vi "Initialise From Font.vi"(7 "Renderer":u32, 8 "Wrap Length [pixels]":i32, 9 "Colour":u32(colorbox), 10 "Text":string, 11 "Font Pointer":u32 format="%.0x") -> (3 "Texture out":refnum<class "Texture.lvclass">)   [LabVIEW 2021, in "Texture.lvclass"]
uses:
  Texture.lvclass
  Texture.lvclass/Texture.ctl
  LabSDL2/Source/Libraries/LibSDL2_TTF Wrapper/LibSDL2_TTF.lvlib
  LabSDL2/Source/Libraries/LibSDL2 Wrapper/LibSDL2.lvlib
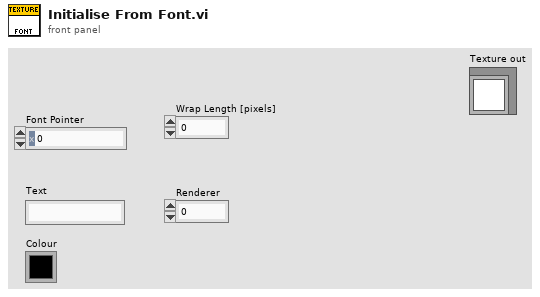
[diagram p1: front panel]
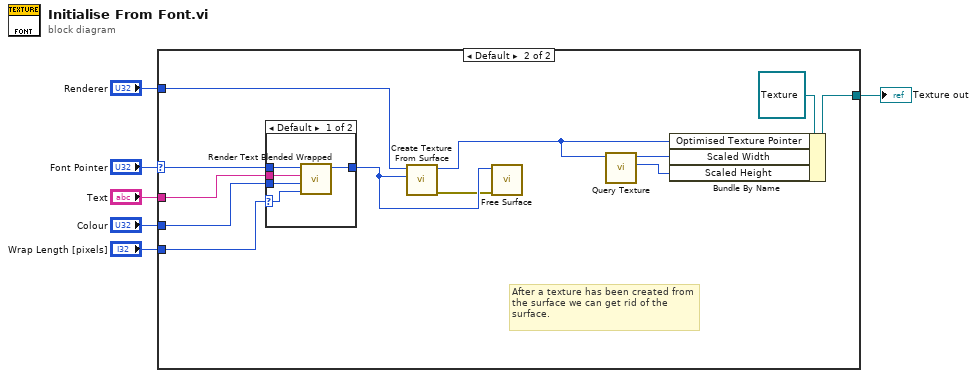
[diagram p0: block diagram]
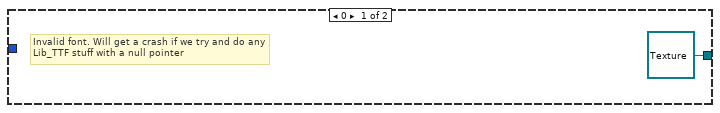
[diagram p2: hidden frame]
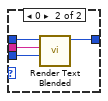
[diagram p3: hidden frame]
diagram:
  n1 = case shown="Default" "Font Pointer" {
    selector: "Font Pointer" -> [_ w16]
    tunnel: [refnum<class "Texture.lvclass"> refnum ("Texture in") w19] -> w6
    tunnel: "Colour" -> [_ w17]
    tunnel: "Text" -> [_ w15]
    tunnel: "Wrap Length [pixels]" -> [_ w9]
    tunnel: "Renderer" -> [_ w8]
    frame 0 {
      # "Invalid font. Will get a crash if we try and do any Lib_TTF stuff with a null pointer"
    }
    frame Default {
      # "After a texture has been created from the surface we can get rid of the surface."
      n2 = case shown="Default" w9 {
        selector: w9 -> [w20 _]
        tunnel: w17 -> [w21 w28]
        tunnel: w16 -> [w23 w27]
        tunnel: w15 -> [w22 w26]
        tunnel: [w24 w25] -> w14
        frame Default {
          n3 = call "Render Text Blended Wrapped.vi"("Length"=w20, "Colour"=w21, "Text"=w22, "Font Pointer"=w23) -> ("Surface Pointer"=w24:u32)  [unwired: 7 in]
        }
        frame 0 {
          n4 = call "Render Text Blended.vi"("Colour"=w28, "Text"=w26, "Font Pointer"=w27) -> ("Surface Pointer"=w25:u32)  [unwired: 8 in]
        }
      }
      n5 = call "Create Texture From Surface.vi"("Surface Pointer"=w14, "Renderer Pointer"=w8) -> ("error out"=w10:errorcluster, "Texture Pointer"=w13:u32)  [unwired: 8 in]
      n6 = call "Free Surface.vi"("error in"=w10, "Surface Pointer"=w14) -> ()  [unwired: 9 in, 1 out]
      n7 = call "Query Texture.vi"("Texture Pointer"=w13) -> ("Height"=w11:i32, "Width"=w12:i32)  [unwired: 7 in, 2 out]
      n8 = Bundle By Name(cluster=refnum<class "Texture.lvclass"> refnum ("Texture in"), "Optimised Texture Pointer"=w13, "Scaled Width"=w12, "Scaled Height"=w11) -> (w19:refnum<class "Texture.lvclass">)
    }
  }
  "Texture out" <- w6
